vi "GetWyPts_enum.vi"(8 "error in (no error)":errorcluster, 11 "Enum":variant) -> (0 "error out":errorcluster, 1 "WyPts":string[](array[string]), 2 "Cmd Number":string, 3 "WyPtFullNode":T1, 4 "found":bool)   [LabVIEW 2020, in "WyPtDict.lvlib"]
doc: "Developed by Kevin Thompson\nkevin@thompsonengineering.net\n\nCopyright 2021\nThompson Engineering, LLC"
uses:
  WyPtDict.lvlib
  support/MC and Robo Handshake.ctl
  RoboWaypointDict Node--cluster.ctl
  WyPtFullNode--cluster.ctl
  StockerExpansionModuleID--enum.ctl
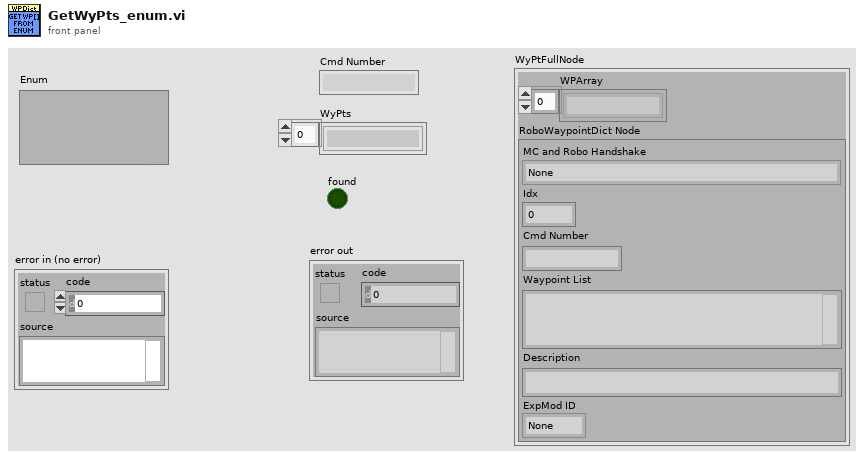
[diagram p1: front panel]
types:
  T1 = typedef "WyPtDict.lvlib/WyPtFullNode--cluster.ctl" = cluster{"WPArray":string[], "RoboWaypointDict Node":T2}
  T2 = typedef "WyPtDict.lvlib/RoboWaypointDict Node--cluster.ctl" = cluster{"MC and Robo Handshake":T3, "Idx":i32, "Cmd Number":string, "Waypoint List":string, "Description":string, "ExpMod ID":T4}
  T3 = typedef "MC and Robo Handshake.ctl" = enum16{"None", "Move and Pick Nikon Ret LP(1100)", "Nikon Barcode1 Scanning Started(1101)", "Nikon Barcode1 Scan Abort(1102)", "Nikon Barcode1 Scan Success Proc to Barcode 2 Pos(1103)", "Nikon Barcode 2 Scanning Started(1104)", "Nikon Barcode 2 Scan Abort(1105) ", "Nikon Barcode 2 Success(1106)", "Move and Pick POZZ Ret LP(1300)", "POZZ Barcode Scan Started(1301)", "POZZ Barcode Not Found(1302)", "POZZ Barcode Scan Succ(1303)", "POZZ Mov to Side 2 Bar 2(1310)", "POZZ Mov to Side 4 Bar 1(1311)", "POZZ Mov to Side 4 Bar 2(1312)", "POZZ Mov to Side 1 Bar 1(1313)", "POZZ Mov to Side 1 Bar 2(1314)", "POZZ Mov to Side 3 Bar 1(1315)", "POZZ Mov to Side 3 Bar 2(1316)", "POZZ Mov to Edge 3 Nik 2(1317)", "POZZ Mov to Edge 4 ASML(1318)", "POZZ Mov to Edge 4 Nik 1(1319)", "POZZ Mov to Edge 4 Nik 2(1320)", "Move to ASML LP and Pick Ret(2000)", "ASML1 Barcode Scan Started(2001)", "ASML1 Barcode Not Found(2002)", "ASML1 Barcode Scan Succ(2003)", "Start Load Seq for Nikon LP(3000)", "Start Load Seq for POZZ LP(3200)", "Start Load Seq for ASML LP(3400)", "Start Align End Grip Place Func(4000)", "Start Align End grip Pick Func(4001)", "Start Align Center Grip Place Func(4002)", "Start Align Center grip Pick Func(4003)", "Start Move from home to Cleaner(5000)", "Start Move to Final Cleaner Loc(5001)", "Start Move from Cleaner loc to home(5002)", "Start Move from home to PDS for Inspect(6000) ", "PDS Inspect Finished(6001)", "PDS EMO Recovery(6002)", "Store in Stocker(7001)", "Store in Expansion Stocker(7402)", "Retrive from Center Stocker(8001)", "Retrive Mov to Nikon BC1 Scan Pos(8002)", "Retrive Nikon BC1not found(8003)", "Retrive Nikon BC1 Scan Succ(8004)", "Retrive Nikon BC2 not found(8005)", "Retrive Nikon BC2 scan Succ(8006)", "Retrive Mov to Edge 1 ASML(8202) ", "Retrive Mov to Edge 1 Nikon 1(8203)", "Retrive Mov to Edge 1 Nikon 2(8204)", "Retrive Mov to Edge 2 ASML(8205)", "Retrive Mov to Edge 2 Nikon 1(8206)", "Retrive Mov to Edge 2 Nikon 2(8207)", "Retrive Mov to Edge 3 ASML (8208)", "Retrive Mov to Edge 3 Nikon 1(8209)", "Retrive Mov to Edge 3 Nikon 2(8210)", "Retrive Mov to Edge 4 ASML (8211)", "Retrive Mov to Edge 4 Nikon 1 (8212)", "Retrive Mov to Edge 4 Nikon 2 (8213)", "Retrive BC Scan Abort (8214)", "Retrive BC Scan Successful (8215)", "Retrive Mov to ASML BC scan Pos (8402) ", "Retrive ASML BC not found(8403)", "Retrive ASML BC Scan Succ(8404)", "Expansion Retrive Seq (8602)", "Cen Stocker move from home to Transit Nest(9000)", "Cen Stocker move from Transit Nest to home(9200)", "Exp Stocker move from home to Transit Nest(9400)", "Exp Stocker move from Transit Nest to home(9600)", "Move to R1 Home (1000)", "Move to R2 Home (1111)", "Store Left Stocker (7401)", "Retrieve Left Stocker (8601)", "EMO Recovery Center (1002)", "EMO Recovery Right (1003)", "Center Robo Status (8888)", "Right Robo Status (8889)"}
  T4 = typedef "WyPtDict.lvlib/StockerExpansionModuleID--enum.ctl" = enum16{"None", "Main", "Exp1", "Exp2", "Exp3", "Exp4", "Exp5"}
  T5 = typedef "Type Descriptor Enumeration__ogtk.ctl" = enum8{"<Null>", "I8", "I16", "I32", "I64", "U8", "U16", "U32", "U64", "SGL", "DBL", "EXT", "CSG", "CDB", "CXT", "0x0F", "0x10", "0x11", "0x12", "0x13", "0x14", "Enum U8", "Enum U16", "Enum U32", "Enum U64", "SGL PQ", "DBL PQ", "EXT PQ", "CSG PQ", "CDB PQ", "CXT PQ", "0x1F", "0x20", "Boolean", "0x22", "0x23", "0x24", "0x25", "0x26", "0x27", "0x28", "0x29", "0x2A", "0x2B", "0x2C", "0x2D", "0x2E", "0x2F", "String", "0x31", "Path", "Pict", "0x34", "0x35", "0x36", "DAQ", "0x38", "0x39", "0x3A", "0x3B", "0x3C", "0x3D", "0x3E", "0x3F", "Array", "0x41", "0x42", "0x43", "0x44", "0x45", "0x46", "0x47", "0x48", "0x49", "0x4A", "0x4B", "0x4C", "0x4D", "0x4E", "0x4F", "Cluster", "0x51", "0x52", "Variant", "Waveform", "0x55", "0x56", "0x57", "0x58", "0x59", "0x5A", "0x5B", "0x5C", "0x5D", "0x5E", "0x5F", "0x60", "0x61", "0x62", "0x63", "0x64", "0x65", "0x66", "0x67", "0x68", "0x69", "0x6A", "0x6B", "0x6C", "0x6D", "0x6E", "0x6F", "Refnum"}
  T6 = typedef "TD Dynamic CVT DVR--ref.ctl" = refnum<data-value>
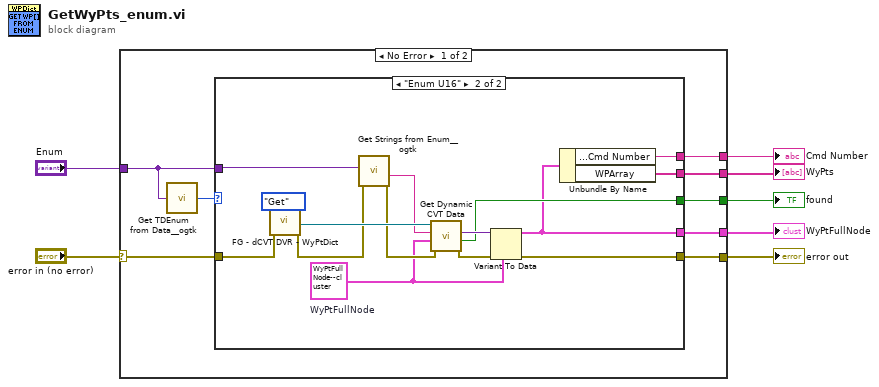
[diagram p0: block diagram]
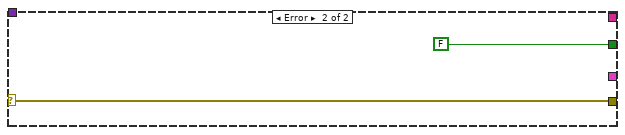
[diagram p3: hidden frame]
diagram:
  n1 = case shown="No Error" "error in (no error)" {
    selector: "error in (no error)" -> [w15 w33]
    tunnel: [w14 w33] -> w7
    tunnel: "Enum" -> [w12 _]
    tunnel: [w11 _] -> w3
    tunnel: [w10 FALSE ("found")] -> w4
    tunnel: [w9 _] -> w2
    tunnel: [w8 _] -> w1
    frame No Error {
      n2 = call <userlib>:"Get TDEnum from Data__ogtk.vi"("Data"=w12) -> ("Type Descriptor Enumeration"=w13:T5)  [unwired: 4 in]
      n3 = case shown="\"Enum U16\"" w13 {
        tunnel: w15 -> [w16 w26]
        tunnel: [w16 w31] -> w14
        tunnel: w12 -> [_ w27]
        tunnel: [_ w19] -> w11
        tunnel: [_ w21] -> w10
        tunnel: [_ w18] -> w9
        tunnel: [_ w17] -> w8
        frame "<Null>", Default {
        }
        frame "Enum U16" {
          w20 = T1 {"WPArray"=[], "RoboWaypointDict Node"={"MC and Robo Handshake"=enum."None", "Idx"=0, "Cmd Number"="", "Waypoint List"="", "Description"="", "ExpMod ID"=enum."None"}}  # WyPtFullNode
          n4 = call "FG - dCVT DVR - WyPtDict.vi"("error in (no error)"=w26, "Action (Get)"=enum16{"Init", "Get", "Set"}."Get") -> ("dCVT WyPt out"=w29:T6, "error out"=w28:errorcluster)  [unwired: 7 in]
          n5 = call <userlib>:"Get Strings from Enum__ogtk.vi"("error in (no error)"=w28, "Enum"=w27) -> ("error out"=w22:errorcluster, "String Value"=w23:string)  [unwired: 6 in, 2 out]
          n6 = call <vilib>:"Get Dynamic CVT Data.vi"("error in (no error)"=w22, "default value (empty variant)"=w20, "DataName"=w23, "dCVT DVR"=w29) -> ("error out"=w25:errorcluster, "found"=w21:bool, "value"=w24:variant)  [unwired: 4 in, 1 out]
          n7 = Variant To Data(error in=w25, type=w20, Variant=w24) -> (data=w19:T1, error out=w31:errorcluster)
          n8 = Unbundle By Name(w19) -> ("RoboWaypointDict Node.Cmd Number"=w17:string, "WPArray"=w18:string[])
        }
      }
    }
    frame Error {
    }
  }
  "error out" <- w7
  "WyPts" <- w2
  "found" <- w4
  "WyPtFullNode" <- w3
  "Cmd Number" <- w1
